vi "2过0法多周期平均子程序.vi"(1 "波形":waveform(dbl)) -> (0 "f":dbl)   [LabVIEW 2017]
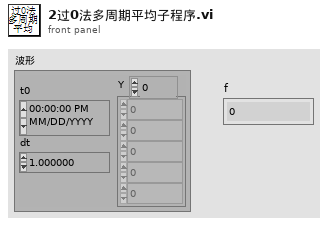
[diagram p1: front panel]
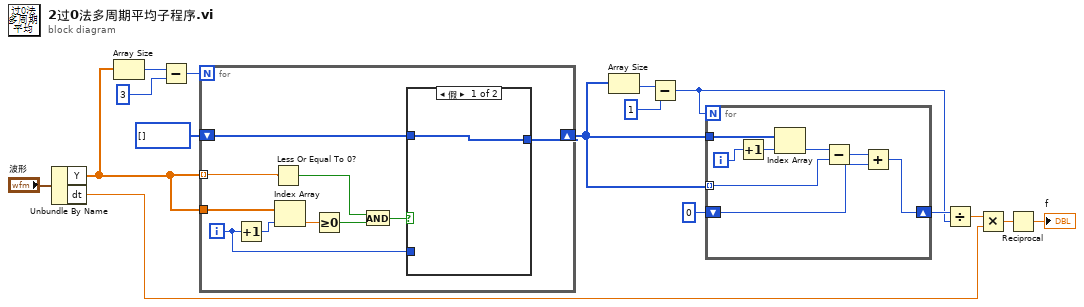
[diagram p0: block diagram]
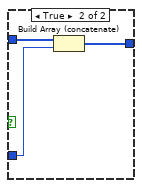
[diagram p2: hidden frame]
diagram:
  n1 = Unbundle By Name("波形") -> ("Y"=w6:dbl[], "dt"=w1:dbl)
  n2 = Array Size(array=w6) -> (size(s)=w8:i32)
  n3 = Subtract(x=w8, y=3) -> (x-y=w5:i32)
  n4 = for {
    N: w5 -> [_]
    tunnel: w6 -> [w23] mode=indexing
    tunnel: w6 -> [w26]
    shift-right: [w17] -> w11
    shift-left: i32[] [] -> [w18]
    i -> [w19]
    n5 = Increment(x=w19) -> (x+1=w25:i32)
    n6 = Less Or Equal To 0?(x=w23) -> (x <= 0?=w21:bool)
    n7 = Index Array(array=w26, index=w25) -> (element=w24:dbl)
    n8 = Greater Or Equal To 0?(x=w24) -> (x >= 0?=w22:bool)
    n9 = And(x=w21, y=w22) -> (x .and. y?=w20:bool)
    n10 = case shown="假" w20 {
      tunnel: w19 -> [_ w30]
      tunnel: w18 -> [w27 w28]
      tunnel: [w27 w29] -> w17
      frame False {
      }
      frame True {
        n11 = Build Array (concatenate)(w28, w30) -> (w29:i32[])
      }
    }
  }
  n12 = Array Size(array=w11) -> (size(s)=w3:i32)
  n13 = Subtract(x=w3, y=1) -> (x-y=w2:i32)
  n14 = for {
    N: w2 -> [_]
    tunnel: w11 -> [w34] mode=indexing
    tunnel: w11 -> [w38]
    shift-right: [w31] -> w10
    shift-left: 0 -> [w32]
    i -> [w37]
    n15 = Increment(x=w37) -> (x+1=w36:i32)
    n16 = Index Array(array=w38, index=w36) -> (element=w35:i32)
    n17 = Subtract(x=w35, y=w34) -> (x-y=w33:i32)
    n18 = Add(x=w33, y=w32) -> (x+y=w31:i32)
  }
  n19 = Divide(x=w10, y=w2) -> (x/y=w9:dbl)
  n20 = Multiply(x=w9, y=w1) -> (x*y=w13:dbl)
  n21 = Reciprocal(x=w13) -> (1/x=→"f":dbl)
